vi "Get_Init_States.vi"(0 "Filename (.ini)":string="Config_Ver_1\\pulse_sequence.ini", 1 "error in":errorcluster) -> (2 "register 1 (2-7)":T2, 3 "register 2 (8-13)":T1, 4 "error out":errorcluster)   [LabVIEW 2021]
uses:
  Drivers/Arduino_Pulse_Generator/Configurate/Register_1.ctl
  Drivers/Arduino_Pulse_Generator/Configurate/Register_2.ctl
  <vilib>/Utility/config.llb/Read Key (Boolean).vi
  <vilib>/Utility/config.llb/NI_LVConfig.lvlib
panel:
  # "Remember that config files are .ini, \nconfig file will be save in ...\\Config_Files\\(filename).ini"
  # "One can easily add files into folder placed inside ...\\Config_Files\\ (folder)\nby writing Filename as (folder)\\(filename).ini, but firstly one have to manualy\ncreate that folder"
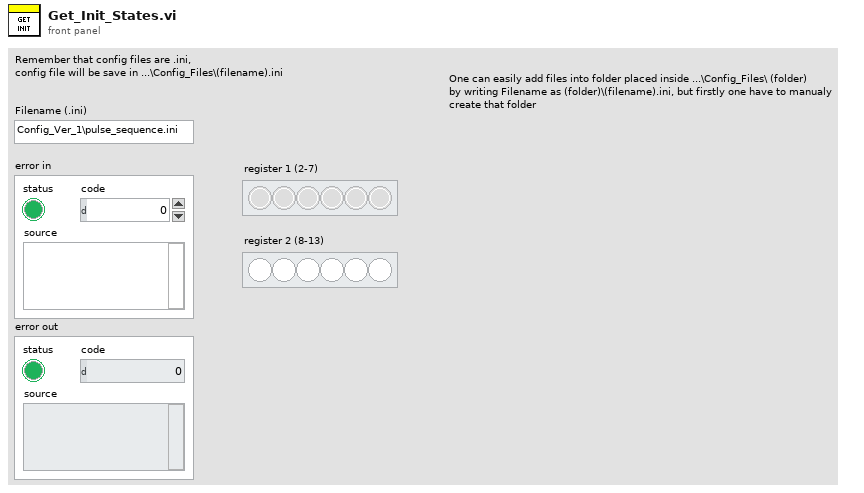
[diagram p1: front panel]
types:
  T1 = typedef "Register_2.ctl" = bool[]
  T2 = typedef "Register_1.ctl" = bool[]
  T3 = typedef "NI_LVConfig.lvlib/Config Data RefNum.ctl" = refnum<k1>
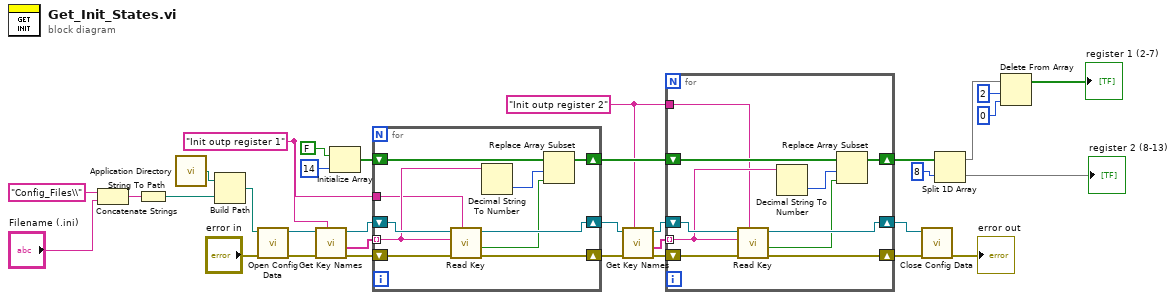
[diagram p0: block diagram]
diagram:
  w4 = "Init outp register 2" ("section")
  w3 = "Init outp register 1" ("section")
  n1 = Concatenate Strings("Config_Files\\" ("string"), "Filename (.ini)") -> (w26:string)
  n2 = String To Path(string=w26) -> (path=w30:path)
  n3 = call <vilib>:"Application Directory.vi"() -> ("Application Directory"=w33:path)
  n4 = Build Path(base path=w33, name or relative path=w30) -> (appended path=w32:path)
  n5 = call <vilib>:"Open Config Data.vi"("error in (no error)"="error in", "configuration file path"=w32) -> ("error out"=w24:errorcluster, "refnum"=w29:T3)  [unwired: 7 in, 1 out]
  n6 = call <vilib>:"Get Key Names.vi"("section"=w3, "error in (no error)"=w24, "refnum"=w29) -> ("error out"=w19:errorcluster, "key names"=w23:string[], "refnum out"=w20:T3)  [unwired: 5 in, 1 out]
  n7 = Initialize Array(FALSE, 14 ("dimension size")) -> (w18:bool[])
  n8 = for {
    tunnel: w23 -> [w40] mode=indexing
    shift-right: [w35] -> w16
    shift-left: w19 -> [w42]
    shift-right: [w41] -> w17
    shift-left: w20 -> [w43]
    shift-right: [w36] -> w12
    shift-left: w18 -> [w38]
    tunnel: w3 -> [w34]
    n9 = call-poly <vilib>:"Read Key.vi"("section"=w34, "error in (no error)"=w42, "key"=w40, "refnum"=w43) -> ("error out"=w35:errorcluster, "value"=w39:bool, "refnum out"=w41:T3)  [unwired: 4 in, 1 out]
    n10 = Decimal String To Number(string=w40) -> (number=w37:i32)  [unwired: 2 in, 1 out]
    n11 = Replace Array Subset(array=w38, new element=w39, index=w37) -> (w36:bool[])
  }
  n12 = call <vilib>:"Get Key Names.vi"("section"=w4, "error in (no error)"=w16, "refnum"=w17) -> ("error out"=w13:errorcluster, "key names"=w14:string[], "refnum out"=w15:T3)  [unwired: 5 in, 1 out]
  n13 = for {
    tunnel: w14 -> [w50] mode=indexing
    shift-right: [w45] -> w5
    shift-left: w13 -> [w52]
    shift-right: [w51] -> w6
    shift-left: w15 -> [w53]
    shift-right: [w46] -> w11
    shift-left: w12 -> [w48]
    tunnel: w4 -> [w44]
    n14 = call-poly <vilib>:"Read Key.vi"("section"=w44, "error in (no error)"=w52, "key"=w50, "refnum"=w53) -> ("error out"=w45:errorcluster, "value"=w49:bool, "refnum out"=w51:T3)  [unwired: 4 in, 1 out]
    n15 = Decimal String To Number(string=w50) -> (number=w47:i32)  [unwired: 2 in, 1 out]
    n16 = Replace Array Subset(array=w48, new element=w49, index=w47) -> (w46:bool[])
  }
  n17 = call <vilib>:"Close Config Data.vi"("error in (no error)"=w5, "refnum"=w6) -> ("error out"=→"error out":errorcluster)  [unwired: 8 in, 1 out]
  n18 = Split 1D Array(array=w11, index=8) -> (first subarray=w9:bool[], second subarray=→"register 2 (8-13)":bool[])
  n19 = Delete From Array(array=w9, length=2, index=0) -> (array with subset deleted=→"register 1 (2-7)":bool[])  [unwired: 1 out]
